vi "Step Time.vi"(6 "Loop Data in":T1, 11 "Sequence in":refnum<class "Sequence.lvclass">) -> (4 "Loop Data":T1)   [LabVIEW 2023, in "VolatusSeq.lvlib" / "Sequence.lvclass"]
uses:
  Sequence.lvclass
  Sequence.lvclass/Sequence.ctl
  Sequence Time.ctl
  VolatusSeq.lvlib
  State/State.lvclass
  Loop Data.ctl
  Volatus/MessageQ/MessageQ.lvclass
  VolatusSeqConfig/Debug Flags.ctl
  VolatusSeqConfig/VolatusSeqConfig.lvlib
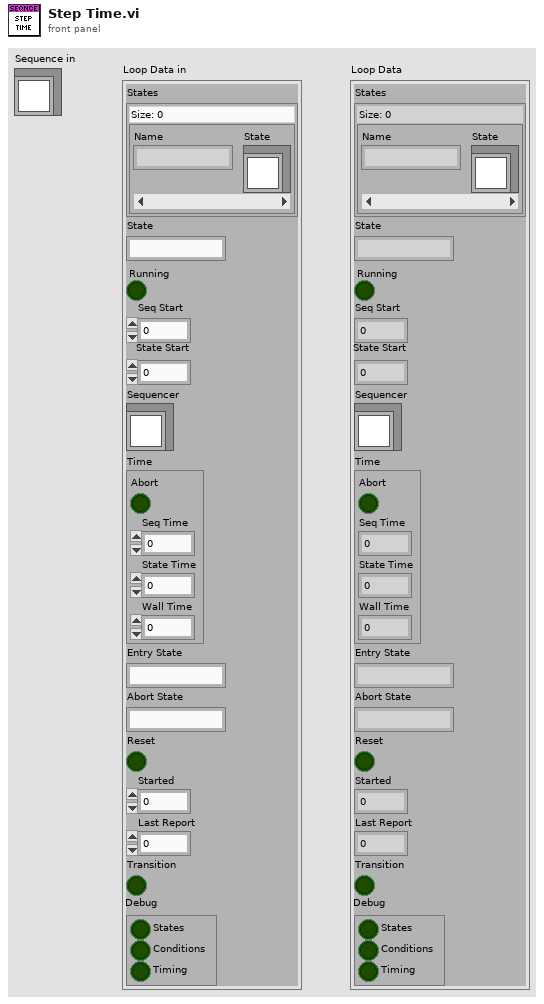
[diagram p1: front panel]
types:
  T1 = typedef "VolatusSeq.lvlib/Sequence.lvclass/Loop Data.ctl" = cluster{"States":map{string, refnum<class "State.lvclass">}, "State":string, "Running":bool, "Seq Start":dbl, "State Start":dbl, "Sequencer":refnum<class "MessageQ.lvclass">, "Time":T2, "Entry State":string, "Abort State":string, "Reset":bool, "Started":dbl, "Last Report":dbl, "Transition":bool, "Debug":T3}
  T2 = typedef "VolatusSeq.lvlib/Sequence Time.ctl" = cluster{"Abort":bool, "Seq Time":dbl, "State Time":dbl, "Wall Time":dbl}
  T3 = typedef "VolatusSeqConfig.lvlib/Debug Flags.ctl" = cluster{"States":bool, "Conditions":bool, "Timing":bool}
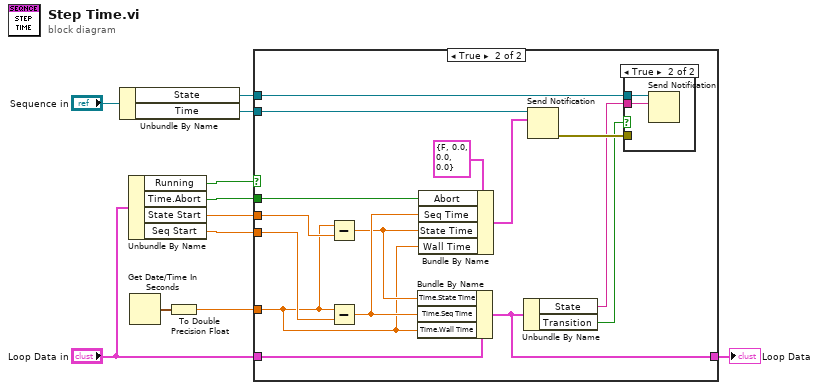
[diagram p0: block diagram]
diagram:
  n1 = Unbundle By Name("Sequence in") -> ("State"=w1:refnum<notifier>, "Time"=w10:refnum<notifier>)
  n2 = Unbundle By Name("Loop Data in") -> ("Running"=w2:bool, "Time.Abort"=w5:bool, "State Start"=w4:dbl, "Seq Start"=w7:dbl)
  n3 = Get Date/Time In Seconds() -> (seconds since 1Jan1904=w9:timestamp)
  n4 = To Double Precision Float(number=w9) -> (double precision float=w3:dbl)
  n5 = case shown="True" w2 {
    tunnel: w10 -> [_ w26]
    tunnel: "Loop Data in" -> [w12 w24]
    tunnel: w7 -> [_ w23]
    tunnel: [w12 w16] -> w6
    tunnel: w5 -> [_ w20]
    tunnel: w4 -> [_ w19]
    tunnel: w3 -> [_ w17]
    tunnel: w1 -> [_ w15]
    frame False {
    }
    frame True {
      n6 = Subtract(x=w17, y=w19) -> (x-y=w18:dbl)
      n7 = Subtract(x=w17, y=w23) -> (x-y=w21:dbl)
      n8 = Bundle By Name(cluster=w24, "Time.State Time"=w18, "Time.Seq Time"=w21, "Time.Wall Time"=w17) -> (w16:T1)
      n9 = Bundle By Name(cluster=T2 {"Abort"=FALSE, "Seq Time"=0.0, "State Time"=0.0, "Wall Time"=0.0} ("notification"), "Abort"=w20, "Seq Time"=w21, "State Time"=w18, "Wall Time"=w17) -> (w22:T2)
      n10 = Unbundle By Name(w16) -> ("State"=w13:string, "Transition"=w14:bool)
      n11 = Send Notification(notification=w22, notifier=w26) -> (error out=w27:errorcluster)  [unwired: 1 in, 1 out]
      n12 = case shown="True" w14 {
        tunnel: w15 -> [_ w29]
        tunnel: w13 -> [_ w28]
        tunnel: w27 -> [_ _]
        frame False {
        }
        frame True {
          n13 = Send Notification(notification=w28, notifier=w29) -> ()  [unwired: 1 in, 2 out]
        }
      }
    }
  }
  "Loop Data" <- w6
